vi "MoveBySteps.vi"(0 "TranslationStage in":refnum<class "BPC30x.lvclass">, 1 "Direction":enum16{"Forward", "Backwards"}(ring)=enum."Backwards", 5 "Steps":dbl, 7 "Channel":u16(ring)=1 items=["Channel1"=1, "Channel2"=2, "Channel3"=3, "Channel4"=4], 9 "Speed":u32, 11 "error in (no error)":errorcluster, 13 "Polarity":enum16{"Positive", "Negative"}(ring)) -> (4 "TranslationStage out":refnum<class "BPC30x.lvclass">, 15 "error out":errorcluster)   [LabVIEW 2023, in "BPC30x.lvlib" / "BPC30x.lvclass"]
uses:
  BPC30x.lvclass
  C:/Program Files/National Instruments/LabVIEW 2023/vi.lib/ActorFramework/Actor/Actor.lvclass
  UIs/TranslationStage_UI/TranslationStage_UI/StageMoveDone_For_UI.ctl
  BPC30x.lvclass/BPC30x.ctl
  <vilib>/ActorFramework/Actor/Actor.lvclass/Actor.ctl
  Interfaces/AbstractInstrumentClasses/TranslationStages_LV/TranslationStagesComm Messages/StageMoveDone Msg/StageMoveDone Msg.lvclass/StageMoveDone Msg.ctl
  <vilib>/ActorFramework/Message Enqueuer/Message Enqueuer.lvclass/Message Enqueuer.ctl
  <vilib>/ActorFramework/Message Enqueuer/Enqueue.vi
  Interfaces/AbstractInstrumentClasses/TranslationStages_LV/TranslationStagesComm Messages/StageMoveDone Msg/StageMoveDone Msg.lvclass
  C:/Program Files/National Instruments/LabVIEW 2023/vi.lib/ActorFramework/Message/Message.lvclass
  C:/Users/quantum/Documents/LVDAQ/Thorlabs.MotionControl.Benchtop.PiezoCLI.dll
  Thorlabs.MotionControl.Benchtop.PiezoCLI.dll
  <vilib>/ActorFramework/Message Priority Queue/Priority Enqueue.vi
  <vilib>/ActorFramework/Actor/Actor.lvclass
  typedefs/typedefs.lvlib
panel:
  in  "Positions":T1={"CH1 Pos"=0.0, "CH2 Pos"=0.0, "CH3 Pos"=0.0, "CH4 Pos"=0.0, "Home?"=TRUE}
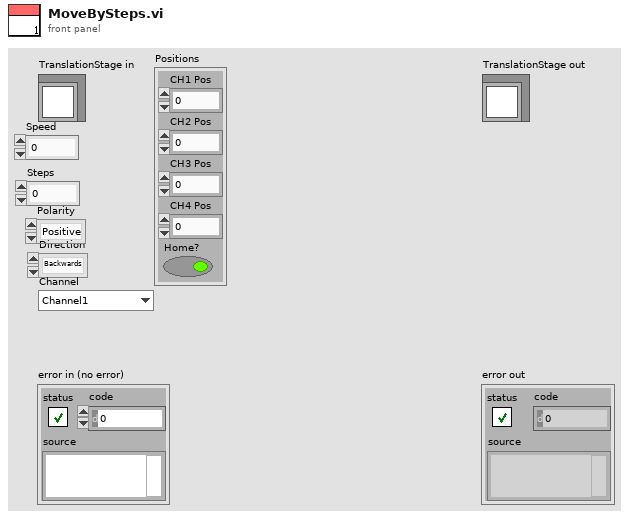
[diagram p1: front panel]
types:
  T1 = typedef "typedefs.lvlib/StageMoveDone_For_UI.ctl" = cluster{"CH1 Pos":sgl, "CH2 Pos":dbl, "CH3 Pos":dbl, "CH4 Pos":dbl, "Home?":bool}
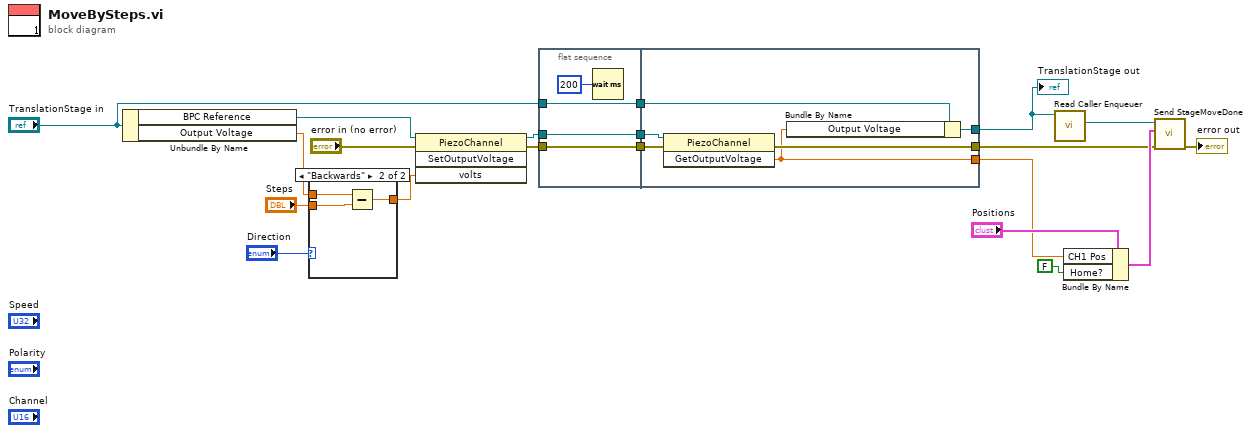
[diagram p0: block diagram]
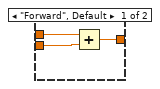
[diagram p2: hidden frame]
diagram:
  n1 = Unbundle By Name("TranslationStage in") -> ("BPC Reference"=w11:refnum<k24>, "Output Voltage"=w9:dbl)
  n2 = case shown="\"Backwards\"" "Direction" {
    tunnel: w9 -> [w23 w26]
    tunnel: "Steps" -> [w22 w25]
    tunnel: [w21 w24] -> w2
    frame "Forward", Default {
      n3 = Add(x=w23, y=w22) -> (x+y=w21:dbl)
    }
    frame "Backwards" {
      n4 = Subtract(x=w26, y=w25) -> (x-y=w24:dbl)
    }
  }
  n5 = invoke class="PiezoChannel" method="SetOutputVoltage"(reference=w11, error in="error in (no error)", "volts"=w2) -> (reference out=w13:refnum<k24>, error out=w16:errorcluster)  [unwired: 1 in, 2 out]
  n6 = flat-sequence {
    tunnel: w13 -> [w28]
    tunnel: "TranslationStage in" -> [w29]
    tunnel: w16 -> [w30]
    tunnel: [w30] -> w5
    tunnel: [w29] -> w4
    tunnel: [w28] -> w3
    tunnel: [w35] -> w14
    tunnel: [w31] -> w6
    tunnel: w5 -> [w33]
    tunnel: w4 -> [w36]
    tunnel: w3 -> [w34]
    tunnel: [w32] -> w1
    frame #0 {
      n7 = Wait (ms)(milliseconds to wait=u32 200) -> ()  [unwired: 1 out]
    }
    frame #1 {
      n8 = invoke class="PiezoChannel" method="GetOutputVoltage"(reference=w34, error in=w33) -> (error out=w32:errorcluster, "GetOutputVoltage"=w31:dbl)  [unwired: 1 in, 1 out]
      n9 = Bundle By Name(cluster=w36, "Output Voltage"=w31) -> (w35:refnum<class "BPC30x.lvclass">)
    }
  }
  n10 = call <vilib>:"Read Caller Enqueuer.vi"("Actor"=w14) -> ("Caller Enqueuer"=w20:refnum<class "Message Enqueuer.lvclass">)  [unwired: 10 in]
  n11 = Bundle By Name(cluster="Positions", "CH1 Pos"=w6, "Home?"=FALSE) -> (w18:T1)
  n12 = call "Send StageMoveDone.vi"("error in (no error)"=w1, "Positions"=w18, "Message Enqueuer"=w20) -> ("error out"=→"error out":errorcluster)  [unwired: 7 in, 1 out]
  "TranslationStage out" <- w14
